vi "test.vi"() -> ()   [LabVIEW 2013]
uses:
  Multiplexer_Opmux.lvclass
panel:
  in  "Command":enum16{"SA", "SI", "SL", "ST", "CT"}(ring)
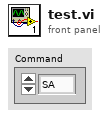
[diagram p1: front panel]
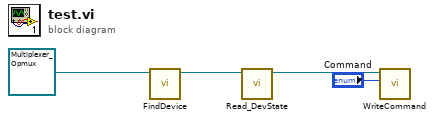
[diagram p0: block diagram]
diagram:
  n1 = call-dynamic "FindDevice.vi"("Multiplexer_Opmux in"=refnum<class "Multiplexer_Opmux.lvclass"> refnum ("Multiplexer_Opmux.lvclass")) -> ("Multiplexer_Opmux out"=w3:refnum<class "Multiplexer_Opmux.lvclass">)  [unwired: 9 in, 1 out]
  n2 = call-dynamic "Read_DevState.vi"("Multiplexer_Opmux in"=w3) -> ("Multiplexer_Opmux out"=w2:refnum<class "Multiplexer_Opmux.lvclass">)  [unwired: 8 in, 2 out]
  n3 = call-dynamic "WriteCommand.vi"("Command"="Command", "Multiplexer_Opmux in"=w2) -> ()  [unwired: 8 in, 2 out]
